vi "GEOM_VAR_OverrideWCS.vi"(9 "Action":T1, 10 "override headers":string[][](array[string]), 11 "override headers mext":string[][][](array[string])) -> (2 "override headers out":string[][](array[string]), 3 "override mext":string[][][](array[string]))   [LabVIEW 2016]
uses:
  GEOM_VAR_action.ctl
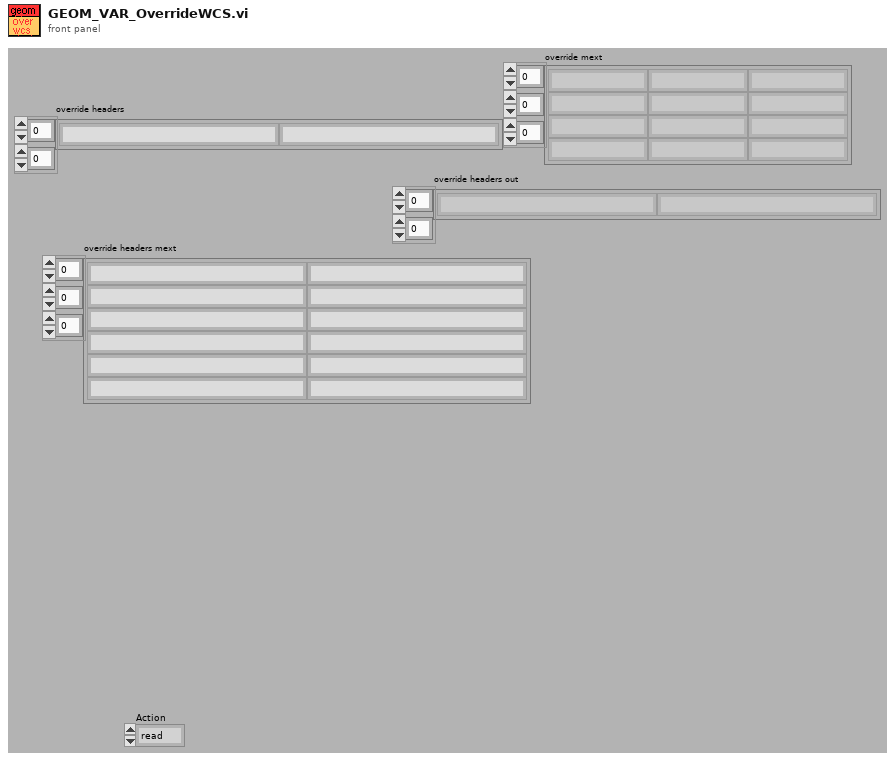
[diagram p1: front panel]
types:
  T1 = typedef "GEOM_VAR_action.ctl" = enum16{"read", "write"}
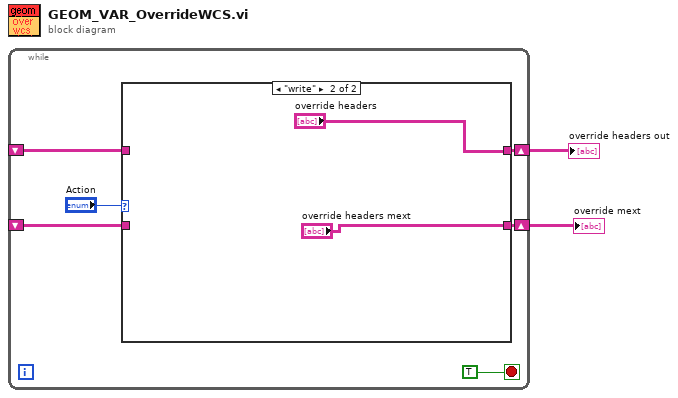
[diagram p0: block diagram]
diagram:
  n1 = while {
    shift-right: [w7] -> w2
    shift-left: _ -> [w6]
    shift-right: [w4] -> w1
    shift-left: _ -> [w3]
    stop <- TRUE stop-if-true
    n2 = case shown="\"write\"" "Action" {
      tunnel: [w10 "override headers"] -> w7
      tunnel: w6 -> [w10 _]
      tunnel: [w9 "override headers mext"] -> w4
      tunnel: w3 -> [w9 _]
      frame "read", Default {
      }
      frame "write" {
      }
    }
  }
  "override headers out" <- w2
  "override mext" <- w1
